vi "Get Pump Voltage.vi"(8 "error in":errorcluster, 11 "CPC in":refnum<class "CPC.lvclass">) -> (0 "error out":errorcluster, 2 "pumpV":dbl, 3 "CPC out":refnum<class "CPC.lvclass">)   [LabVIEW 2014, in "CPC.lvclass"]
doc: "The value retrieved with the command is 0-10 V with 0 representing 1.55 V and 10 representing 12 V to the pump."
uses:
  CPC.lvclass
  Controls/3022A/Enum Cmd.ctl
  3022A/3022A.lvclass
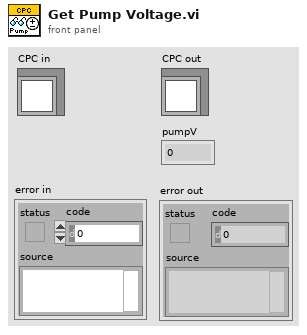
[diagram p1: front panel]
types:
  T1 = typedef "3022A.lvclass/Enum Cmd.ctl" = enum8{"CALIBRATE", "GET CAL DATA", "DUMP", "ESCAPE", "ID CAL LABEL", "INPUT CAL LABEL", "LIQUID LEVEL", "CONDENSER T", "SATURATOR T", "OPTICS T", "GET FLOW RATE", "READ ENV", "READ REF DETECTOR", "READ DETECTOR V", "READ 200 s BUFFER", "READ 20 s BUFFER", "READ 2 s BUFFER", "READ 1 s BUFFER", "READ PHOTOMETRIC CONC", "READ FP CONC", "READ MICROPROCESSOR PUMP CTL", "SENSOR", "SET VOLTAGE", "WRITE DISP MSG", "LASER OFF", "LASER ON", "PUMP OFF", "PUMP ON", "DRAIN", "FILL", "RESET CONC BUFFERS", "LOW FLOW MODE", "HIGH FLOW MODE"}
  T2 = cluster{"Cmd":T1, "x":i64, "y":i64, "Display":string}
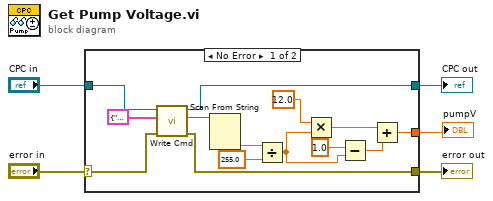
[diagram p0: block diagram]
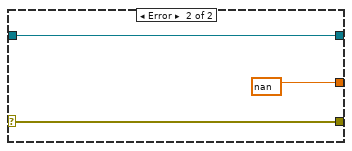
[diagram p2: hidden frame]
diagram:
  n1 = case shown="No Error" "error in" {
    selector: "error in" -> [w19 w22]
    tunnel: [w18 w22] -> w4
    tunnel: [w16 w21] -> w2
    tunnel: "CPC in" -> [w17 w21]
    tunnel: [w11 nan] -> w1
    frame No Error {
      n2 = call-dynamic "Write Cmd.vi"("error in"=w19, "CmdStruct"=T2 {"Cmd"=enum."READ MICROPROCESSOR PUMP CTL", "x"=0, "y"=0, "Display"=""}, "CPC in"=w17) -> ("error out"=w18:errorcluster, "Buffer"=w14:string, "CPC out"=w16:refnum<class "CPC.lvclass">)  [unwired: 6 in]
      n3 = Scan From String(input string=w14) -> (output 1=w8:dbl)  [unwired: 4 in, 3 out]
      n4 = Divide(x=w8, y=255.0) -> (x/y=w6:dbl)
      n5 = Multiply(x=12.0, y=w6) -> (x*y=w9:dbl)
      n6 = Subtract(x=1.0, y=w6) -> (x-y=w10:dbl)
      n7 = Add(x=w9, y=w10) -> (x+y=w11:dbl)
    }
    frame Error {
    }
  }
  "error out" <- w4
  "CPC out" <- w2
  "pumpV" <- w1
